vi "ButtonPressCounter.vi"() -> ()   [LabVIEW 2020]
panel:
  in  "stop 2":bool
  out "Count 2":u16
  in  "Ok 2":bool
  in  "stop":bool
  out "Count":u16
  in  "Ok":bool
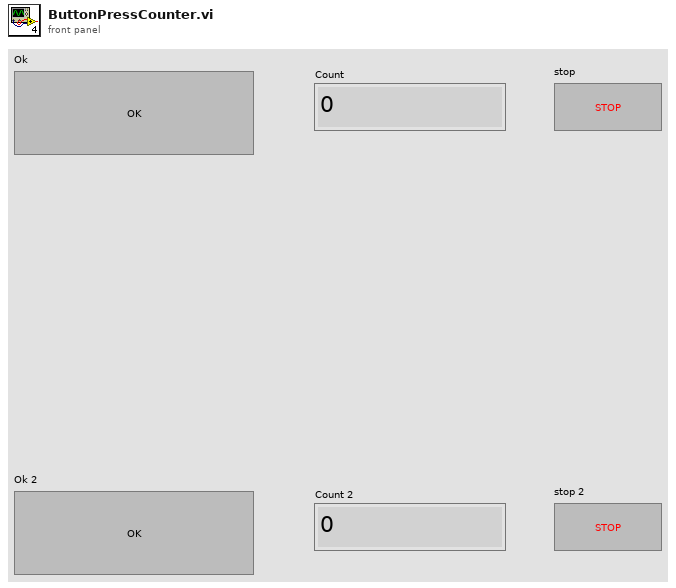
[diagram p1: front panel]
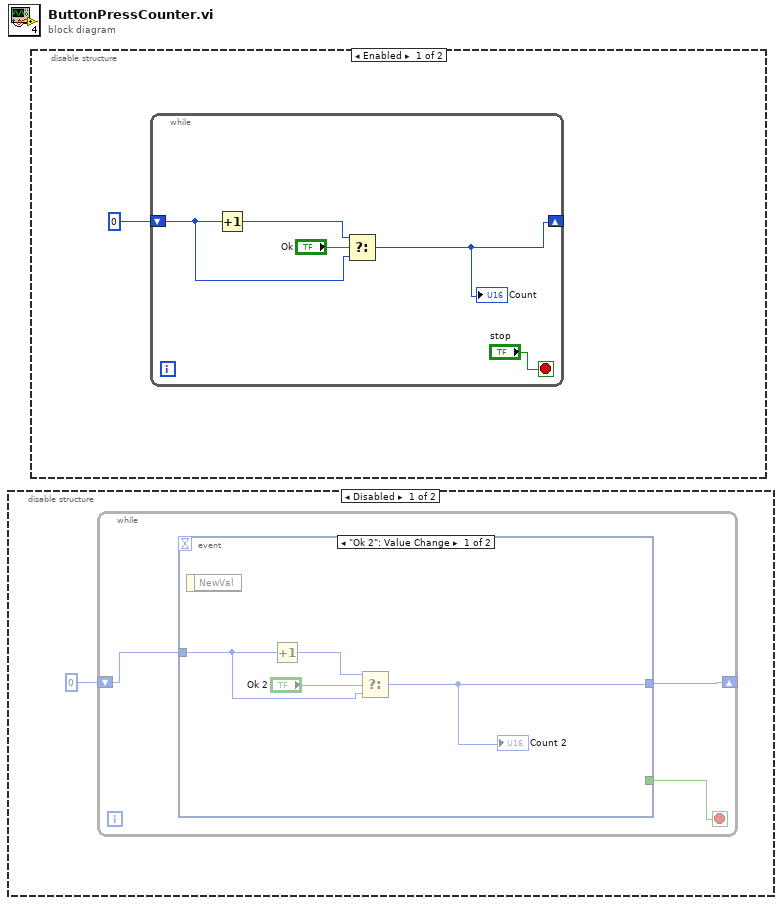
[diagram p0: block diagram]
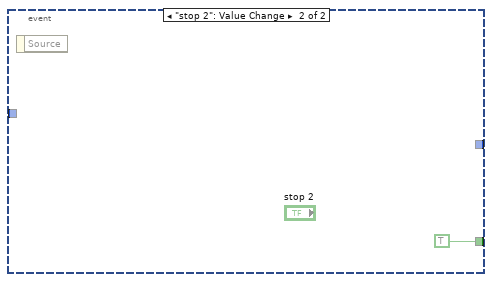
[diagram p2: hidden frame]
diagram:
  n1 = disable-structure shown="Disabled" {
    frame Disabled {
      n2 = while {
        shift-right: [w3] -> _
        shift-left: u16 0 ("Count 2") -> [w4]
        stop <- w2 stop-if-true
        n3 = event shown="[0] \"Ok 2\": Value Change" {
          selector: _ -> [_ _]
          dyn-events: _ -> [_ _]
          timeout: _ -> [_ _]
          tunnel: w4 -> [w6 _]
          tunnel: [w5 _] -> w3
          tunnel: [_ TRUE] -> w2
          event "Ok 2": Value Change {
            n4 = event-data() -> ()  [unwired: 1 in, 1 out]
            n5 = Increment(x=w6) -> (x+1=w7:u16)
            n6 = Select(t=w7, s="Ok 2", f=w6) -> (s? t:f=w5:u16)
            "Count 2" <- w5
          }
          event "stop 2": Value Change {
            n7 = event-data() -> ()  [unwired: 1 in, 1 out]
          }
        }
      }
    }
    frame Enabled {
    }
  }
  n8 = disable-structure shown="Enabled" {
    frame Enabled {
      n9 = while {
        shift-right: [w12] -> _
        shift-left: u16 0 ("Count") -> [w13]
        stop <- "stop" stop-if-true
        n10 = Increment(x=w13) -> (x+1=w14:u16)
        n11 = Select(t=w14, s="Ok", f=w13) -> (s? t:f=w12:u16)
        "Count" <- w12
      }
    }
    frame Disabled {
    }
  }
